vi "ABB Test Noise.vi"() -> ()   [LabVIEW 2017]
uses:
  <vilib>/Analysis/baseanly.llb/Mean (DBL).vi
  ABB global.vi
  <vilib>/Analysis/NI_AALBase.lvlib
panel:
  in  "Case Constant\n(See Context Help)":bool=TRUE
  in  "Octave analysis":bool
  in  "Specified Noise":dbl
  in  "Noise Limit":dbl
  in  "Number Points":i32
  out "Noise During Run dB(A)":dbl format="%#.1g"
  out "Noise Before Run dB(A)":dbl format="%#.1g"
  in  "Motor Type":u16(ring) items=["horizontal motor", "vertical motor", "12 points"]
  out "Picture":picture
  in  "Noise levels dB(A)":string[][](table)
  out "Serial number":string
  out "W.O number":string
  out "Timedate":string
  in  "Exit":bool
  # "Noise levels"
  # "?"
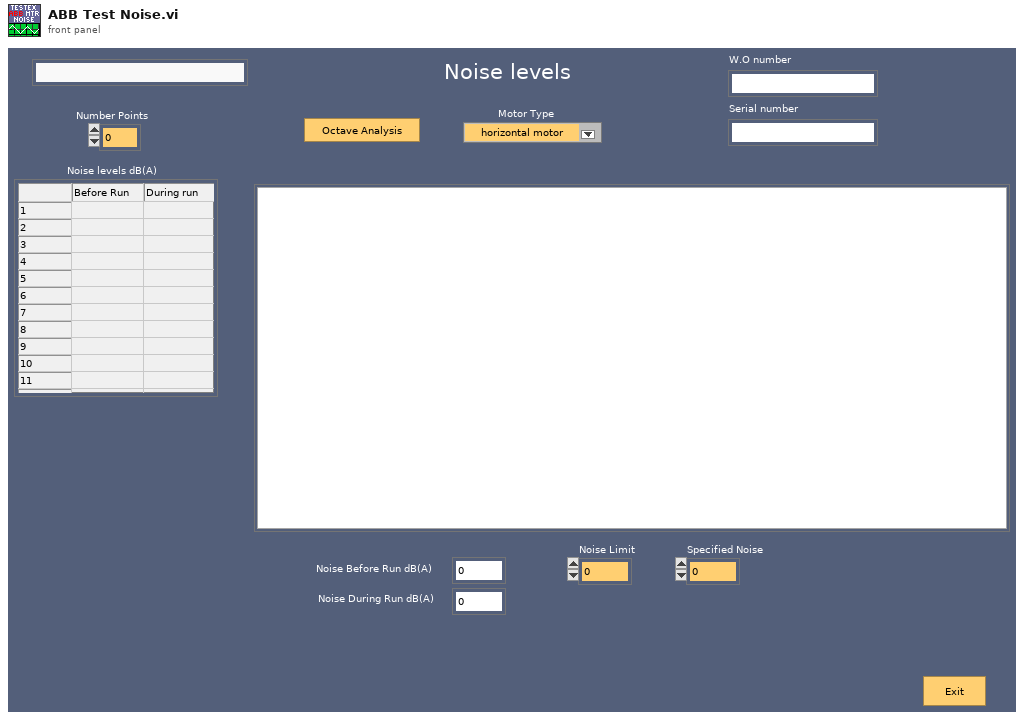
[diagram p1: front panel]
types:
  T1 = cluster{"integer":i32, "Dbl":dbl, "String":string, "Boolean":bool}
  T2 = cluster{"Simulate Norma":bool, "Norma 5000 Address":u8, "WebDaq IP Address":string, "Simulate cDAQ":bool}
  T3 = typedef "imagedata.ctl" = cluster{"image type":i32, "image depth":i32, "image":u8[], "mask":u8[], "colors":u32[], "Rectangle":cluster{"left":i16, "top":i16, "right":i16, "bottom":i16}}
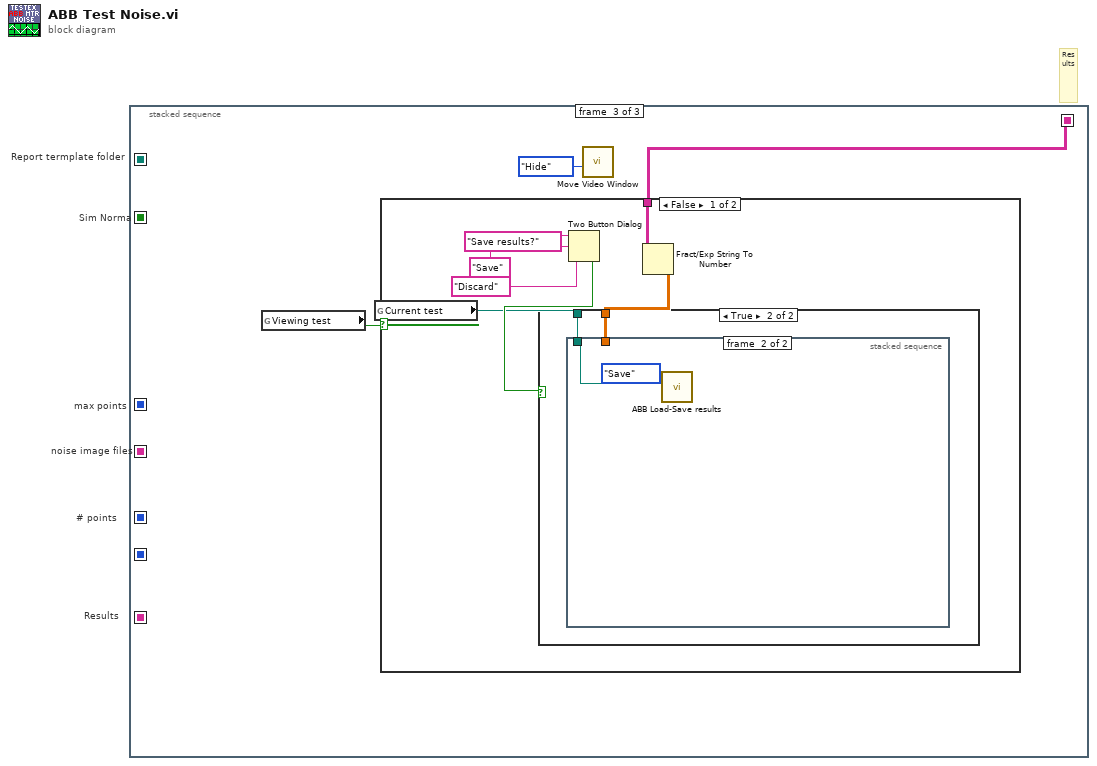
[diagram p0: block diagram]
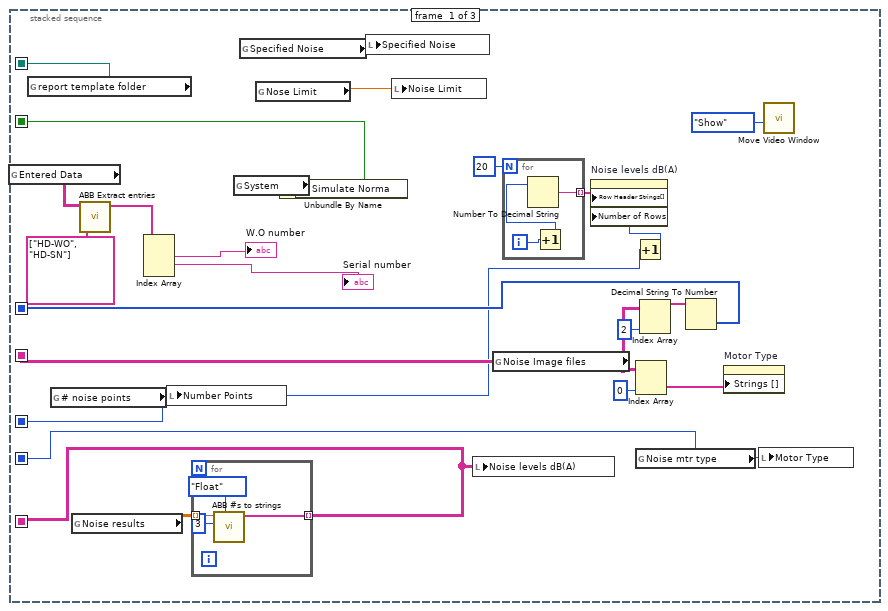
[diagram p2: hidden frame]
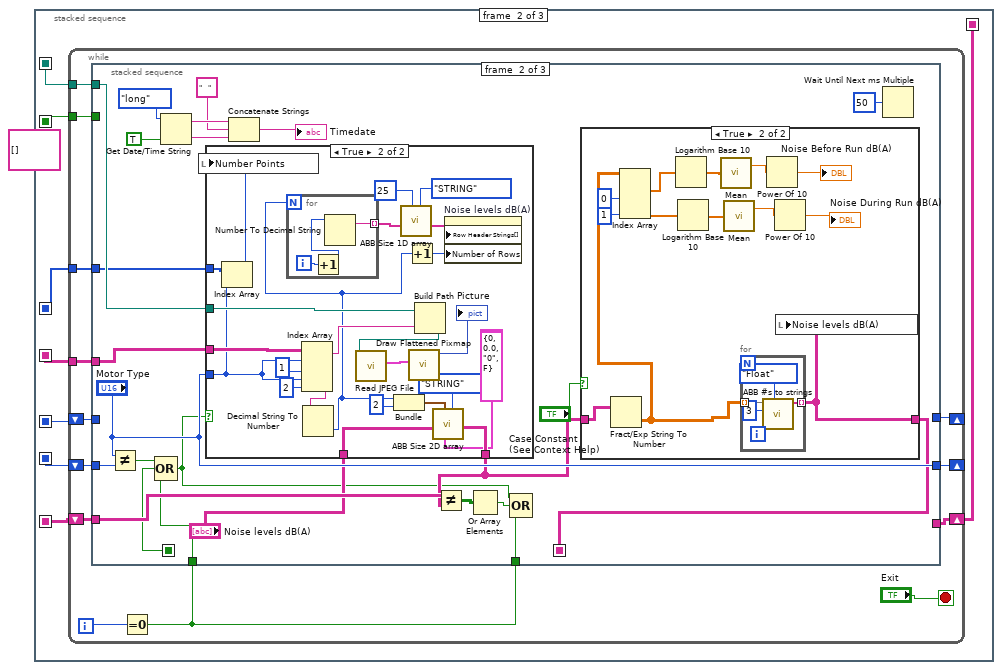
[diagram p3: hidden frame]
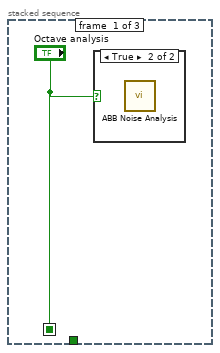
[diagram p4: hidden frame]
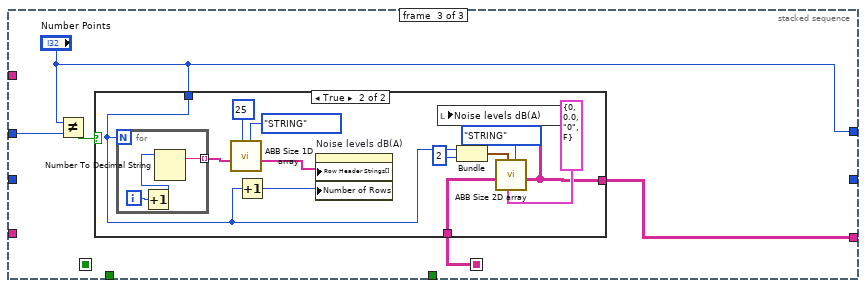
[diagram p8: hidden frame]
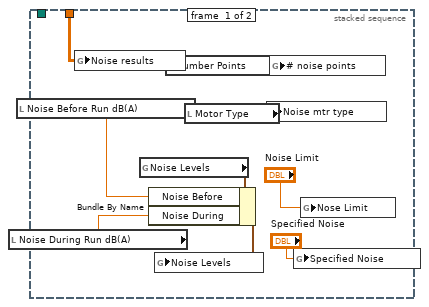
[diagram p11: hidden frame]
diagram:
  # "# points"
  # "max points"
  # "Report termplate folder"
  # "Sim Norma"
  # "Results"
  # "noise image files"
  # "Results"
  n1 = stacked-sequence {
    seq-local: [w23 _ _] -> [_ w39 _]
    seq-local: [w11 _ _] -> [_ w36 _]
    seq-local: [_ w35 _] -> [_ _ w146]
    seq-local: [w10 _ _] -> [_ w38 _]
    seq-local: [w13 _ _] -> [_ w37 _]
    seq-local: [w7 _ _] -> [_ w34 _]
    seq-local: [w6 _ _] -> [_ w33 _]
    seq-local: [w4 _ _] -> [_ w32 _]
    frame #0 {
      n2 = global read "ABB global.vi" "Entered Data"() -> (w20:string[][])
      n3 = global read "ABB global.vi" "report template folder"() -> (w13:path)
      n4 = global read "ABB global.vi" "# noise points"() -> (w6:i32)
      n5 = global read "ABB global.vi" "Noise results"() -> (w12:dbl[][])
      n6 = call "ABB Extract entries.vi"("Entry IDs"=string[] ["HD-WO", "HD-SN"], "Entry table in"=w20) -> ("Selected Entries"=w19:string[])  [unwired: 9 in]
      n7 = Index Array(array=w19) -> (element #1=→"W.O number":string, element #2=→"Serial number":string)  [unwired: 3 in, 1 out]
      n8 = local write "Number Points"(w6) -> ()
      n9 = for {
        tunnel: w12 -> [w28] mode=indexing
        tunnel: [w25] -> w11 mode=indexing
        n10 = call "ABB #s to strings.vi"("# type"=enum16{"Float", "Relative time HH:MM"}."Float", "Precision"=3, "Numbers in"=w28) -> ("Strings out"=w25:string[])  [unwired: 8 in]
      }
      n11 = global read "ABB global.vi" "System"() -> (w24:T2)
      n12 = global read "ABB global.vi" "Specified Noise"() -> (w2:dbl)
      n13 = global read "ABB global.vi" "Nose Limit"() -> (w3:dbl)
      n14 = Unbundle By Name(w24) -> ("Simulate Norma"=w23:bool)
      n15 = local write "Specified Noise"(w2) -> ()
      n16 = local write "Noise Limit"(w3) -> ()
      n17 = local write "Noise levels dB(A)"(w11) -> ()
      n18 = global read "ABB global.vi" "Noise Image files"() -> (w10:string[][])
      n19 = for {
        N: 20 -> [_]
        tunnel: [w29] -> w21 mode=indexing
        i -> [w31]
        n20 = Increment(x=w31) -> (x+1=w30:i32)
        n21 = Number To Decimal String(number=w30) -> (decimal integer string=w29:string)  [unwired: 1 in]
      }
      n22 = Increment(x=w6) -> (x+1=w5:i32)
      n23 = property on="Noise levels dB(A)" class="Tbl (strict)"("Row Header Strings[]"=w21, "Number of Rows"=w5) -> ()  [unwired: 2 in, 2 out]
      n24 = Index Array(array=w10, index (col)=0 ("disabled index (col)")) -> (element=w14:string[])  [unwired: 1 in]
      n25 = global read "ABB global.vi" "Noise mtr type"() -> (w4:i32)
      n26 = Index Array(array=w10, index (col)=2 ("disabled index (col)")) -> (element=w8:string[])  [unwired: 1 in]
      n27 = Decimal String To Number(string=w8) -> (number=w7:i32[])  [unwired: 2 in, 1 out]
      n28 = property on="Motor Type" class="Ring (strict)"("Strings []"=w14) -> ()  [unwired: 2 in, 2 out]
      n29 = local write "Motor Type"(w4) -> ()
      n30 = call "Move Video Window.vi"("Action"=enum16{"Show", "Hide", "Exit"}."Show") -> ()  [unwired: 11 in]
    }
    frame #1 {
      (unwired) string[][] [] ("Cooling Curve Data")
      n31 = while {
        tunnel: w39 -> [w51]
        shift-right: [w49] -> _
        shift-left: w32 -> [w50]
        tunnel: w38 -> [w48]
        tunnel: w37 -> [w47]
        shift-right: [w42] -> w35
        shift-left: w36 -> [w46]
        tunnel: w34 -> [w45]
        shift-right: [w43] -> _
        shift-left: w33 -> [w44]
        i -> [w41]
        stop <- "Exit" stop-if-true
        n32 = Equal To 0?(x=w41) -> (x = 0?=w40:bool)
        n33 = stacked-sequence {
          seq-local: [_ w60 _] -> [_ _ w125]
          seq-local: ["Octave analysis" _ _] -> [_ w55 _]
          tunnel: w51 -> [_ _ _]
          tunnel: w50 -> [_ w70 _]
          tunnel: [_ "Motor Type" _] -> w49
          tunnel: w48 -> [_ w69 _]
          tunnel: w47 -> [_ w68 _]
          tunnel: [_ _ w124] -> w42
          tunnel: w46 -> [_ w67 _]
          tunnel: w45 -> [_ w61 _]
          tunnel: w44 -> [_ _ w128]
          tunnel: [_ _ "Number Points"] -> w43
          tunnel: w40 -> [_ w59 _]
          tunnel: w40 -> [_ w54 _]
          frame #0 {
            n34 = case shown="True" "Octave analysis" {
              frame False {
              }
              frame True {
                n35 = call "ABB Noise Analysis.vi"() -> ()  [unwired: 6 in]
              }
            }
          }
          frame #1 {
            n36 = Not Equal?(x="Motor Type", y=w70) -> (x != y?=w56:bool)
            n37 = Compound Arithmetic op=OR(w56, w55, w54) -> (w57:bool)
            n38 = Get Date/Time String(date format (0)=enum16{"short", "long", "abbreviated"}."long", want seconds? (F)=TRUE) -> (date string=w75:string, time string=w74:string)  [unwired: 1 in]
            n39 = case shown="True" w57 {
              tunnel: "Motor Type" -> [_ w99]
              tunnel: w69 -> [_ w116]
              tunnel: w68 -> [_ w114]
              tunnel: "Noise levels dB(A)" -> [w96 w111]
              tunnel: [w96 w107] -> w62
              tunnel: w61 -> [_ w98]
              frame False {
              }
              frame True {
                (unwired) T1 {"integer"=0, "Dbl"=0.0, "String"="0", "Boolean"=FALSE} ("Defaults")
                n40 = Index Array(array=w98, index=w99) -> (element=w97:i32)
                n41 = local write "Number Points"(w97) -> ()
                n42 = Index Array(array=w116, index (row) #1=w99, index (col) #1=1 ("disabled index (col)"), index (row) #2=w99, index (col) #2=2 ("disabled index (col)")) -> (element #1=w117:string, element #2=w112:string)
                n43 = Decimal String To Number(string=w112) -> (number=w101:i32)  [unwired: 2 in, 1 out]
                n44 = for {
                  N: w101 -> [_]
                  tunnel: [w121] -> w105 mode=indexing
                  i -> [w123]
                  n45 = Increment(x=w123) -> (x+1=w122:i32)
                  n46 = Number To Decimal String(number=w122) -> (decimal integer string=w121:string)  [unwired: 1 in]
                }
                n47 = Bundle(w101, 2) -> (w109:cluster{i32, i32})  [unwired: 1 in]
                n48 = call "ABB Size 1D array.vi"("Type"=enum16{"Integer", "DBL", "STRING", "BOOLEAN"}."STRING", "Size"=25, "String Array in"=w105) -> ("String Array out"=w104:string[])  [unwired: 5 in, 3 out]
                n49 = Increment(x=w101) -> (x+1=w100:i32)
                n50 = Build Path(base path=w114, name or relative path=w117) -> (appended path=w118:path)
                n51 = call <vilib>:"Read JPEG File.vi"("path to JPEG file"=w118) -> ("image data"=w119:T3)  [unwired: 8 in, 2 out]
                n52 = call <vilib>:"Draw Flattened Pixmap.vi"("image data"=w119) -> ("new picture"=→"Picture":picture)  [unwired: 8 in]
                n53 = call "ABB Size 2D array.vi"("Type"=enum16{"Integer", "DBL", "STRING", "BOOLEAN"}."STRING", "Defaults"=T1 {"integer"=0, "Dbl"=0.0, "String"="0", "Boolean"=FALSE}, "Size"=w109, "String Array in"=w111) -> ("String Array out"=w107:string[][])  [unwired: 4 in, 3 out]
                n54 = property on="Noise levels dB(A)" class="Tbl (strict)"("Row Header Strings[]"=w104, "Number of Rows"=w100) -> ()  [unwired: 2 in, 2 out]
              }
            }
            n55 = Concatenate Strings(w75, "   ", w74) -> (→"Timedate":string)
            n56 = Not Equal?(x=w67, y=w62) -> (x != y?=w66:bool[][])
            n57 = Or Array Elements(Boolean array=w66) -> (logical OR=w65:bool)
            n58 = Compound Arithmetic op=OR(w57, w65, w59) -> ()  [unwired: 1 out]
            n59 = case shown="True" "Case Constant\n(See Context Help)" {
              tunnel: w62 -> [w78 w90]
              tunnel: [w78 w91] -> w60
              frame False {
              }
              frame True {
                n60 = Fract/Exp String To Number(string=w90) -> (number=w89:dbl[][])  [unwired: 3 in, 1 out]
                n61 = Index Array(array=w89, index (col) #1=0 ("disabled index (col)"), index (col) #2=1 ("index (col)")) -> (element #1=w86:dbl[], element #2=w82:dbl[])  [unwired: 2 in]
                n62 = Logarithm Base 10(1:w86) -> (0:w85:dbl[])
                n63 = Logarithm Base 10(1:w82) -> (0:w81:dbl[])
                n64 = call-poly <vilib>:"Mean.vi"("X"=w85) -> ("mean"=w84:dbl)  [unwired: 1 out]
                n65 = call-poly <vilib>:"Mean.vi"("X"=w81) -> ("mean"=w80:dbl)  [unwired: 1 out]
                n66 = for {
                  tunnel: w89 -> [w95] mode=indexing
                  tunnel: [w94] -> w91 mode=indexing
                  n67 = call "ABB #s to strings.vi"("# type"=enum16{"Float", "Relative time HH:MM"}."Float", "Precision"=3, "Numbers in"=w95) -> ("Strings out"=w94:string[])  [unwired: 8 in]
                }
                n68 = Power Of 10(x=w84) -> (10^x=→"Noise Before Run dB(A)":dbl)
                n69 = Power Of 10(x=w80) -> (10^x=→"Noise During Run dB(A)":dbl)
                n70 = local write "Noise levels dB(A)"(w91) -> ()
              }
            }
            n71 = Wait Until Next ms Multiple(millisecond multiple=u32 50) -> ()  [unwired: 1 out]
          }
          frame #2 {
            n72 = Not Equal?(x="Number Points", y=w128) -> (x != y?=w127:bool)
            n73 = case shown="True" w127 {
              tunnel: "Number Points" -> [_ w134]
              tunnel: w125 -> [w129 w132]
              tunnel: [w129 w130] -> w124
              frame False {
              }
              frame True {
                n74 = for {
                  N: w134 -> [_]
                  tunnel: [w142] -> w141 mode=indexing
                  i -> [w144]
                  n75 = Increment(x=w144) -> (x+1=w143:i32)
                  n76 = Number To Decimal String(number=w143) -> (decimal integer string=w142:string)  [unwired: 1 in]
                }
                n77 = call "ABB Size 1D array.vi"("Type"=enum16{"Integer", "DBL", "STRING", "BOOLEAN"}."STRING", "Size"=25, "String Array in"=w141) -> ("String Array out"=w138:string[])  [unwired: 5 in, 3 out]
                n78 = Increment(x=w134) -> (x+1=w137:i32)
                n79 = property on="Noise levels dB(A)" class="Tbl (strict)"("Row Header Strings[]"=w138, "Number of Rows"=w137) -> ()  [unwired: 2 in, 2 out]
                n80 = Bundle("Number Points"=w134, 2) -> (w135:cluster{"Number Points":i32, i32})  [unwired: 1 in]
                n81 = call "ABB Size 2D array.vi"("Type"=enum16{"Integer", "DBL", "STRING", "BOOLEAN"}."STRING", "Defaults"=T1 {"integer"=0, "Dbl"=0.0, "String"="0", "Boolean"=FALSE}, "Size"=w135, "String Array in"=w132) -> ("String Array out"=w130:string[][])  [unwired: 4 in, 3 out]
                n82 = local write "Noise levels dB(A)"(w130) -> ()
              }
            }
          }
        }
      }
    }
    frame #2 {
      n83 = global read "ABB global.vi" "Viewing test"() -> (w147:bool)
      n84 = case shown="False" w147 {
        tunnel: w146 -> [w151 _]
        frame False {
          n85 = global read "ABB global.vi" "Current test"() -> (w152:path)
          n86 = Two Button Dialog(message="Save results?", 1:"Discard" ("F button name (\"Cancel\")"), 2:"Save" ("T button name (\"OK\")")) -> (T button?=w153:bool)
          n87 = Fract/Exp String To Number(string=w151) -> (number=w150:dbl[][])  [unwired: 3 in, 1 out]
          n88 = case shown="True" w153 {
            tunnel: w150 -> [_ w156]
            tunnel: w152 -> [_ w155]
            frame False {
            }
            frame True {
              n89 = stacked-sequence {
                tunnel: w156 -> [w165 _]
                tunnel: w155 -> [_ w166]
                frame #0 {
                  n90 = local read "Noise During Run dB(A)"() -> (w162:dbl)
                  n91 = local read "Noise Before Run dB(A)"() -> (w161:dbl)
                  n92 = global write "ABB global.vi" "Noise results"(w165) -> ()
                  n93 = global read "ABB global.vi" "Noise Levels"() -> (w164:cluster{"Noise Before":dbl, "Noise During":dbl})
                  n94 = Bundle By Name(cluster=w164, "Noise Before"=w161, "Noise During"=w162) -> (w163:cluster{"Noise Before":dbl, "Noise During":dbl})
                  n95 = global write "ABB global.vi" "Noise Levels"(w163) -> ()
                  n96 = local read "Number Points"() -> (w160:i32)
                  n97 = local read "Motor Type"() -> (w159:u16)
                  n98 = global write "ABB global.vi" "Noise mtr type"(w159) -> ()
                  n99 = global write "ABB global.vi" "# noise points"(w160) -> ()
                  n100 = global write "ABB global.vi" "Specified Noise"("Specified Noise") -> ()
                  n101 = global write "ABB global.vi" "Nose Limit"("Noise Limit") -> ()
                }
                frame #1 {
                  n102 = call "ABB Load-Save results.vi"("Path"=w166, "Mode"=enum16{"LOAD", "Save"}."Save") -> ()  [unwired: 10 in]
                }
              }
            }
          }
        }
        frame True {
        }
      }
      n103 = call "Move Video Window.vi"("Action"=enum16{"Show", "Hide", "Exit"}."Hide") -> ()  [unwired: 11 in]
    }
  }
